vi "SubVI_Filter_EEG_NotLossy.vi"(7 "Interpolant Size":dbl, 8 "error in (no error)":errorcluster, 9 "high cutoff freq":dbl, 10 "EEG Desired Frequency":dbl, 11 "Channel in":T1) -> (0 "error out":errorcluster, 3 "Channel out":T1)   [LabVIEW 2020]
uses:
  <extravilib>/ChannelInstances/Stream-a[.,.](dbl)/)Channel.ctl
  <vilib>/Analysis/3filter.llb/Filter Passband Type.ctl
  <extravilib>/ChannelInstances/Stream-a[.,.](dbl)/EndpointRead.vi
  <extravilib>/ChannelInstances/Stream-a[.,.](dbl)/Endpoint.vi
  Global 1.vi
  <extravilib>/ChannelInstances/Stream-a[.,.](dbl)/)Channel.vi
  <resource>/ChannelSupport/_ChannelSupport/WaitIfNeeded.vi
  <vilib>/Analysis/NI_AALBase.lvlib
  <vilib>/ptbypt/NI_PtbyPt.lvlib
  <extravilib>/ChannelInstances/Stream-a[.,.](dbl).lvlib
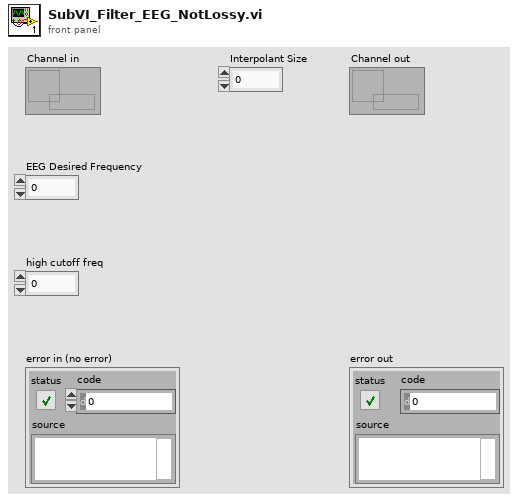
[diagram p1: front panel]
types:
  T1 = typedef "Stream-a[.,.](dbl).lvlib/)Channel.ctl" = refnum<queue>
  T2 = typedef "NI_AALBase.lvlib/Filter Passband Type.ctl" = enum32{"Lowpass", "Highpass", "Bandpass", "Bandstop"}
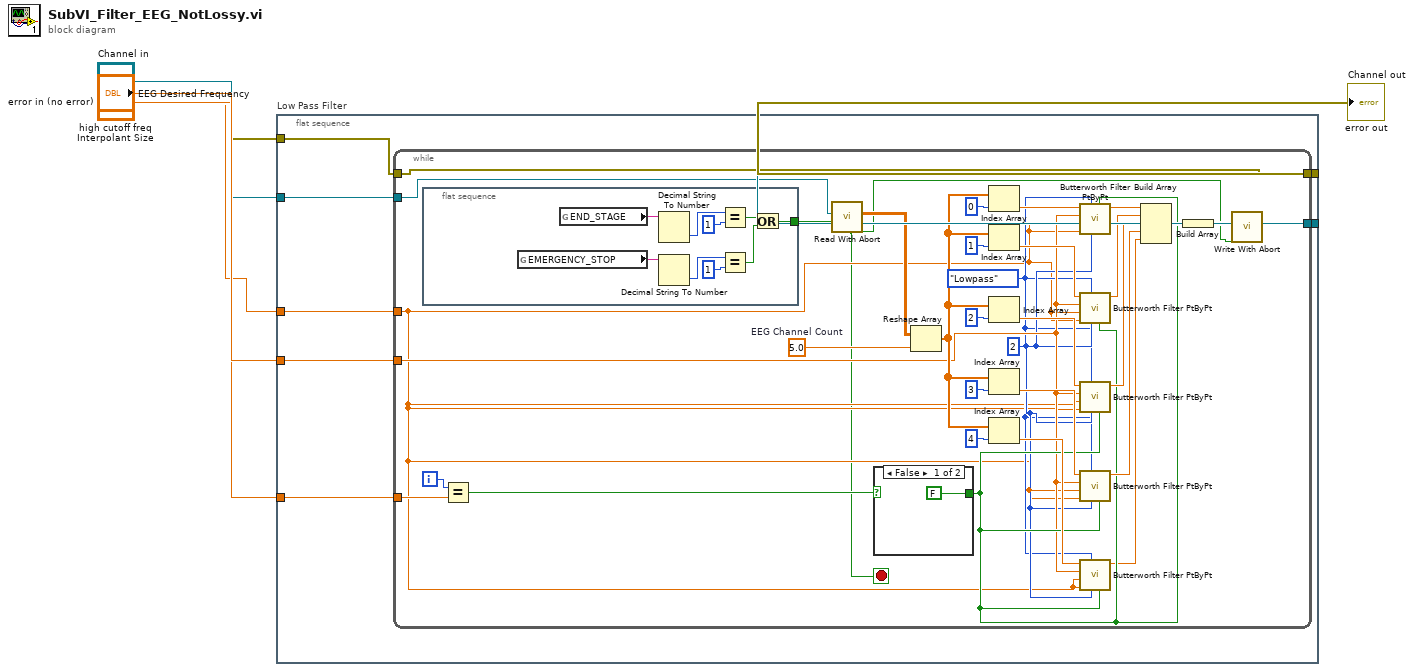
[diagram p0: block diagram]
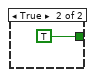
[diagram p2: hidden frame]
diagram:
  n1 = flat-sequence "Low Pass Filter" {
    tunnel: "Channel in" -> [w14]
    tunnel: [w13] -> w3
    tunnel: "Interpolant Size" -> [w12]
    tunnel: "EEG Desired Frequency" -> [w11]
    tunnel: "error in (no error)" -> [w10]
    tunnel: [w9] -> w4
    tunnel: "high cutoff freq" -> [w8]
    frame #0 {
      n2 = while {
        tunnel: w14 -> [w34]
        tunnel: [w15] -> w13
        tunnel: w12 -> [w31]
        tunnel: w11 -> [w25]
        tunnel: w10 -> [w19]
        tunnel: [w19] -> w9
        tunnel: w8 -> [w18]
        i -> [w32]
        stop <- w16 stop-if-true
        w21 = 5.0  # EEG Channel Count
        w24 = 2 ("order")
        w23 = Filter_Passband_Type."Lowpass" ("filter type")
        n3 = flat-sequence {
          tunnel: [w48] -> w20
          frame #0 {
            n4 = global read "Global 1.vi" "EMERGENCY_STOP"() -> (w51:string)
            n5 = global read "Global 1.vi" "END_STAGE"() -> (w56:string)
            n6 = Decimal String To Number(string=w56) -> (number=w55:i32)  [unwired: 2 in, 1 out]
            n7 = Decimal String To Number(string=w51) -> (number=w53:i32)  [unwired: 2 in, 1 out]
            n8 = Equal?(x=w55, y=1) -> (x = y?=w49:bool)
            n9 = Equal?(x=w53, y=1) -> (x = y?=w50:bool)
            n10 = Or(x=w49, y=w50) -> (x .or. y?=w48:bool)
          }
        }
        n11 = Equal?(x=w32, y=w31) -> (x = y?=w30:bool)
        n12 = call <extravilib>:"Read With Abort.vi"("abort"=w20, "channel"=w34) -> ("element"=w33:dbl[][], "aborted?"=w16:bool)  [unwired: 4 in, 4 out]
        n13 = case shown="False" w30 {
          tunnel: [FALSE ("init/cont (init:F)") TRUE ("init/cont (init:F)")] -> w26
          frame False {
          }
          frame True {
          }
        }
        n14 = Reshape Array(w33, w21) -> (w27:dbl[])
        n15 = Index Array(array=w27, index=0 ("disabled index (col)")) -> (element=w43:dbl)
        n16 = Index Array(array=w27, index=1 ("disabled index (col)")) -> (element=w44:dbl)
        n17 = Index Array(array=w27, index=2 ("disabled index (col)")) -> (element=w45:dbl)
        n18 = Index Array(array=w27, index=3 ("disabled index (col)")) -> (element=w46:dbl)
        n19 = Index Array(array=w27, index=4 ("disabled index (col)")) -> (element=w29:dbl)
        n20 = call <vilib>:"Butterworth Filter PtByPt.vi"("initialize"=w26, "order"=w24, "filter type"=w23, "low cutoff freq: fl"=w18, "high cutoff freq: fh"=w18, "sampling freq: fs"=w25, "x"=w43) -> ("Filtered x"=w39:dbl)  [unwired: 2 in, 1 out]
        n21 = call <vilib>:"Butterworth Filter PtByPt.vi"("initialize"=w26, "order"=w24, "filter type"=w23, "low cutoff freq: fl"=w18, "high cutoff freq: fh"=w18, "sampling freq: fs"=w25, "x"=w44) -> ("Filtered x"=w40:dbl)  [unwired: 2 in, 1 out]
        n22 = call <vilib>:"Butterworth Filter PtByPt.vi"("initialize"=w26, "order"=w24, "filter type"=w23, "low cutoff freq: fl"=w18, "high cutoff freq: fh"=w18, "sampling freq: fs"=w25, "x"=w45) -> ("Filtered x"=w41:dbl)  [unwired: 2 in, 1 out]
        n23 = call <vilib>:"Butterworth Filter PtByPt.vi"("initialize"=w26, "order"=w24, "filter type"=w23, "low cutoff freq: fl"=w18, "high cutoff freq: fh"=w18, "sampling freq: fs"=w25, "x"=w46) -> ("Filtered x"=w42:dbl)  [unwired: 2 in, 1 out]
        n24 = call <vilib>:"Butterworth Filter PtByPt.vi"("initialize"=w26, "order"=w24, "filter type"=w23, "low cutoff freq: fl"=w18, "high cutoff freq: fh"=w18, "sampling freq: fs"=w25, "x"=w29) -> ("Filtered x"=w22:dbl)  [unwired: 2 in, 1 out]
        n25 = Build Array(w39, w40, w41, w42, w22) -> (w47:dbl[])
        n26 = Build Array(w47) -> (w17:dbl[][])
        n27 = call <extravilib>:"Write With Abort.vi"("abort"=w16, "element"=w17) -> ("channel"=w15:T1)  [unwired: 6 in, 3 out]
      }
    }
  }
  "error out" <- w4
  "Channel out" <- w3
